vi "Close BreadcrumbNavigator.vi"(8 "error in (no error)":errorcluster, 11 "BreadcrumbNavigation in":refnum<class "BreadcrumbNavigator.lvclass">) -> (0 "error out":errorcluster)   [LabVIEW 2015, in "BreadcrumbNavigator.lvclass"]
doc: "The Deconstructor Method closes the QControl Class and ensures all references are closed. If this method is not used when closing the owning program, the Event Handlers will still be closed but the State Data DVRs and any other references started might not be and cause memory leaks. Best practice would be to use the Deconstructor Method. It is named \"Close\" and then the name of the QControl Class (i.e. Close StatusHistory.vi).\n\nThe Decontructor Method will then:\n1. Call the Close State Data Method\n2. Call the Close Control Method\n<b> </b> <b> </b>\n©2016 Q Software Innovations, LLC (QSI)\nwritten by Quentin Alldredge\nproduced in LabVIEW 2015\n\nsupport@qsoftwareinnovations.com\nwww.qsoftwareinnovations.com\n\nAll rights reserved.\n\nRedistribution and use in source and binary forms, with or without modification, are permitted provided that the following conditions are met:\n\n * Redistributions of source code must retain the above copyright notice, this list of conditions and the following disclaimer.\n * Redistributions in binary form must reproduce the above copyright notice, this list of conditions and the following disclaimer in the documentation and/or other materials provided with the distribution.\n * Neither the name of Q Software Innovations, LLC. nor the names of its contributors may be used to endorse or promote products derived from this software without specific prior written permission.\n\nTHIS SOFTWARE IS PROVIDED BY THE COPYRIGHT HOLDERS AND CONTRIBUTORS \"AS IS\" AND ANY EXPRESS OR IMPLIED WARRANTIES, INCLUDING, BUT NOT LIMITED TO, THE IMPLIED WARRANTIES OF MERCHANTABILITY AND FITNESS FOR A PARTICULAR PURPOSE ARE DISCLAIMED. IN NO EVENT SHALL THE COPYRIGHT OWNER OR CONTRIBUTORS BE LIABLE FOR ANY DIRECT, INDIRECT, INCIDENTAL, SPECIAL, EXEMPLARY, OR CONSEQUENTIAL DAMAGES (INCLUDING, BUT NOT LIMITED TO, PROCUREMENT OF SUBSTITUTE GOODS OR SERVICES; LOSS OF USE, DATA, OR PROFITS; OR BUSINESS INTERRUPTION) HOWEVER CAUSED AND ON ANY THEORY OF LIABILITY, WHETHER IN CONTRACT, STRICT LIABILITY, OR TORT (INCLUDING NEGLIGENCE OR OTHERWISE) ARISING IN ANY WAY OUT OF THE USE OF THIS SOFTWARE, EVEN IF ADVISED OF THE POSSIBILITY OF SUCH DAMAGE."
uses:
  BreadcrumbNavigator.lvclass
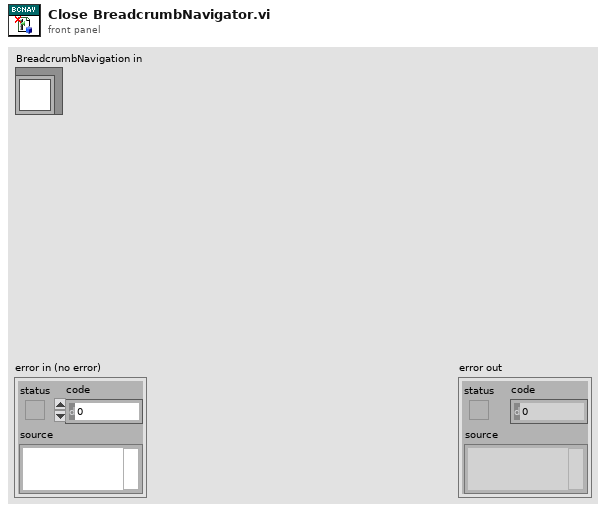
[diagram p1: front panel]
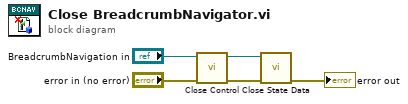
[diagram p0: block diagram]
diagram:
  n1 = call-dynamic "Close Control.vi"("error in (no error)"="error in (no error)", "BreadcrumbNavigation in"="BreadcrumbNavigation in") -> ("error out"=w4:errorcluster, "BreadcrumbNavigation out"=w1:refnum<class "BreadcrumbNavigator.lvclass">)  [unwired: 8 in]
  n2 = call-dynamic "Close State Data.vi"("error in (no error)"=w4, "BreadcrumbNavigation in"=w1) -> ("error out"=→"error out":errorcluster)  [unwired: 8 in, 1 out]
